vi "Motor-Pega-Pos.vi"(0 "MG17Motor 2":refnum<k7>, 1 "error out":errorcluster) -> (2 "MG17Motor 3":refnum<k7>, 3 "pfPosition":sgl, 4 "error out 2":errorcluster)   [LabVIEW 2014]
doc: "André Romero - 2016\nandretec@ifsc.usp.br\nIFSC - USP"
panel:
  out "GetPosition":i32
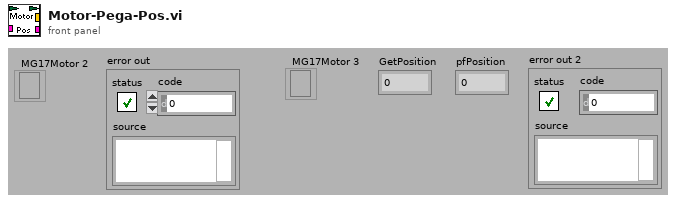
[diagram p1: front panel]
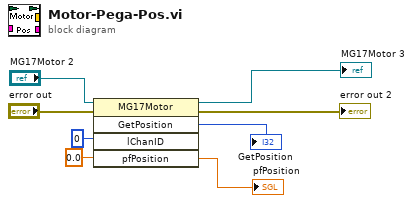
[diagram p0: block diagram]
diagram:
  n1 = invoke class="MG17Motor" method="GetPosition"(reference="MG17Motor 2", error in="error out", "lChanID"=0, "pfPosition"=sgl 0.0) -> (reference out=→"MG17Motor 3":refnum<k7>, error out=→"error out 2":errorcluster, "GetPosition"=→"GetPosition":i32, "pfPosition"=→"pfPosition":sgl)  [unwired: 1 in, 1 out]
